vi "GFITS_LOCKBUF.vi"(8 "error in":errorcluster, 10 "bufname":string) -> (0 "error out":errorcluster, 2 "locked buffer":T1)   [LabVIEW 2016]
uses:
  Common/Clib/lib/libmem.so.20
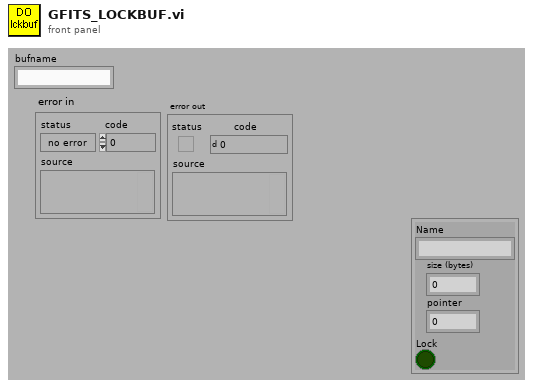
[diagram p1: front panel]
types:
  T1 = cluster{"Name":string, "size (bytes)":u32, "pointer":u32, "Lock":bool}
  T2 = cluster{"Name":string, "size (bytes)":u64, "pointer":u64, "Lock":bool}
  T3 = cluster{"name":string, "Path":path, "bitpix":i8, "naxis":u8, "naxes":u32[], "datatype":u16, "multiple extensions":bool, "hdutype":u16, "writeToDisk":bool, "num_of_ext":u8, "file ref":i32, "createnewimage":bool}
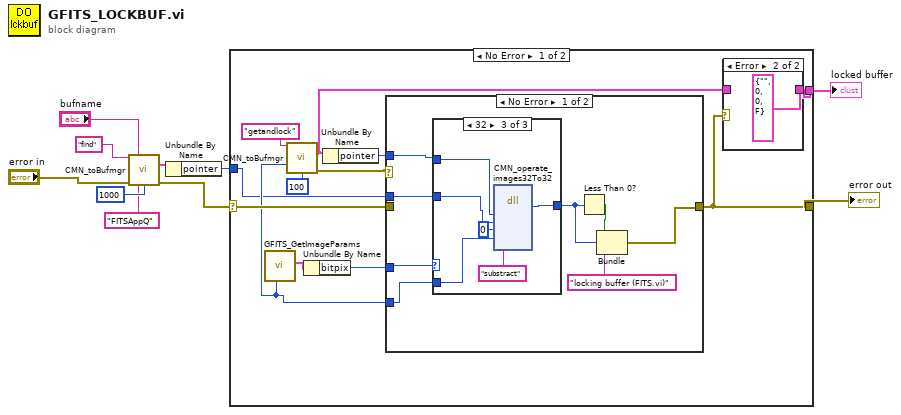
[diagram p0: block diagram]
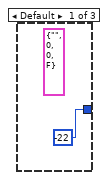
[diagram p3: hidden frame]
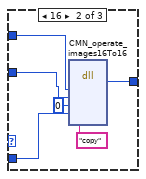
[diagram p4: hidden frame]
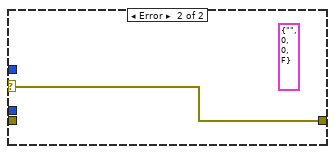
[diagram p5: hidden frame]
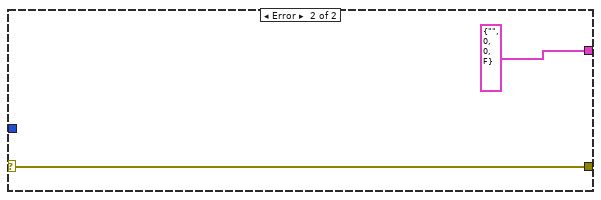
[diagram p6: hidden frame]
diagram:
  n1 = call "CMN_toBufmgr.vi"("command"="find", "bufname"="bufname", "error in"="error in", "responseQ"="FITSAppQ" ("response Q"), "ms timeout (-1)"=1000) -> ("buffer"=w7:T2, "error out"=w6:errorcluster)  [unwired: 3 in, 6 out]
  n2 = Unbundle By Name(w7) -> ("pointer"=w5:u64)
  n3 = case shown="No Error" w6 {
    selector: w6 -> [w16 w48]
    tunnel: [w13 w48] -> w3
    tunnel: w5 -> [w14 _]
    tunnel: [w11 T1 {"Name"="", "size (bytes)"=0, "pointer"=0, "Lock"=FALSE} ("buffer")] -> w1
    frame No Error {
      n4 = call "GFITS_GetImageParams.vi"() -> ("imageStruct"=w20:T3, "totele"=w15:u32)  [unwired: 2 in, 8 out]
      n5 = call "CMN_toBufmgr.vi"("command"="getandlock", "bufsize"=w15, "ms timeout (-1)"=100) -> ("buffer"=w12:T2, "error out"=w19:errorcluster)  [unwired: 5 in, 6 out]
      n6 = Unbundle By Name(w20) -> ("bitpix"=w18:i8)
      n7 = Unbundle By Name(w12) -> ("pointer"=w17:u64)
      n8 = case shown="No Error" w19 {
        selector: w19 -> [_ w46]
        tunnel: w18 -> [w32 _]
        tunnel: w17 -> [w31 _]
        tunnel: w16 -> [_ _]
        tunnel: w15 -> [w30 _]
        tunnel: [w25 w46] -> w13
        tunnel: w14 -> [w29 _]
        frame No Error {
          n9 = case shown="32" w32 {
            tunnel: w30 -> [_ w39 w45]
            tunnel: w31 -> [_ w37 w43]
            tunnel: w29 -> [_ w35 w41]
            tunnel: [-22 w34 w40] -> w27
            frame Default {
              (unwired) T1 {"Name"="", "size (bytes)"=0, "pointer"=0, "Lock"=FALSE} ("buffer")
            }
            frame 16 {
              n10 = dll-call lib="home/simager/panview/PAN/Modules/Common/Clib/lib/libmem.so.20" fn="CMN_operate_images16To16" label="16To16"("image1ptr"=w37, "image2ptr"=w35, "imageptr3"=u64 0, "num_elems"=w39, "operation"="copy") -> ("return type"=w34:i32)  [unwired: 7 in, 3 out]
            }
            frame 32 {
              n11 = dll-call lib="home/simager/panview/PAN/Modules/Common/Clib/lib/libmem.so.20" fn="CMN_operate_images32To32" label="32To32"("image1ptr"=w43, "image2ptr"=w41, "imageptr3"=u64 0, "num_elems"=w45, "operation"="substract") -> ("return type"=w40:i32)  [unwired: 7 in, 3 out]
            }
          }
          n12 = Less Than 0?(x=w27) -> (x < 0?=w28:bool)
          n13 = Bundle(w28, "return type"=w27, "locking buffer (FITS.vi)") -> (w25:cluster{bool, "return type":i32, string})  [unwired: 1 out]
        }
        frame Error {
          (unwired) T1 {"Name"="", "size (bytes)"=0, "pointer"=0, "Lock"=FALSE} ("buffer")
        }
      }
      n14 = case shown="Error" w13 {
        tunnel: w12 -> [w23 _]
        tunnel: [w23 T1 {"Name"="", "size (bytes)"=0, "pointer"=0, "Lock"=FALSE} ("buffer")] -> w11
        frame No Error {
        }
        frame Error {
        }
      }
    }
    frame Error {
    }
  }
  "error out" <- w3
  "locked buffer" <- w1
